vi "WPI_SolenoidSafetyError.vi"(0 "SolenoidDevRef":T1={"DevStatus"={"status"=FALSE, "code"=0, "source"=""}, "Pneumatics Control Module"=1, "Forward Solenoid Channel"=enum."Solenoid 0", "Reverse Solenoid Channel"=enum."Invalid"}) -> (4 "SolenoidDevRef 2":T1={"DevStatus"={"status"=FALSE, "code"=0, "source"=""}, "Pneumatics Control Module"=1, "Forward Solenoid Channel"=enum."Solenoid 0", "Reverse Solenoid Channel"=enum."Invalid"})   [LabVIEW 2017]
doc: "This subVI does two things:\n1. It builds up output specific information to help locate the problem.\n2. It calls the FRC Build Error, so all the information gets passed to the Driver Station."
uses:
  <vilib>/Rock Robotics/WPI/Solenoid/WPI_SolenoidDevRef.ctl
  <vilib>/Rock Robotics/WPI/Solenoid/WPI_SolenoidChannel.ctl
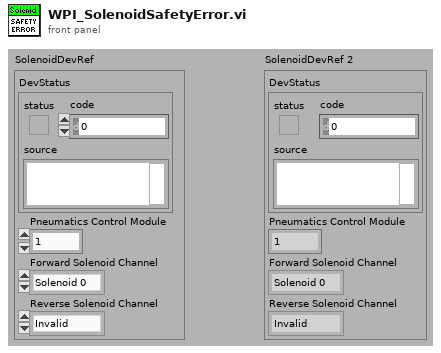
[diagram p1: front panel]
types:
  T1 = typedef "WPI_SolenoidDevRef.ctl" = cluster{"DevStatus":errorcluster, "Pneumatics Control Module":u8, "Forward Solenoid Channel":T2, "Reverse Solenoid Channel":T2}
  T2 = typedef "WPI_SolenoidChannel.ctl" = enum8{"Solenoid 0", "Solenoid 1", "Solenoid 2", "Solenoid 3", "Solenoid 4", "Solenoid 5", "Solenoid 6", "Solenoid 7", "Invalid"}
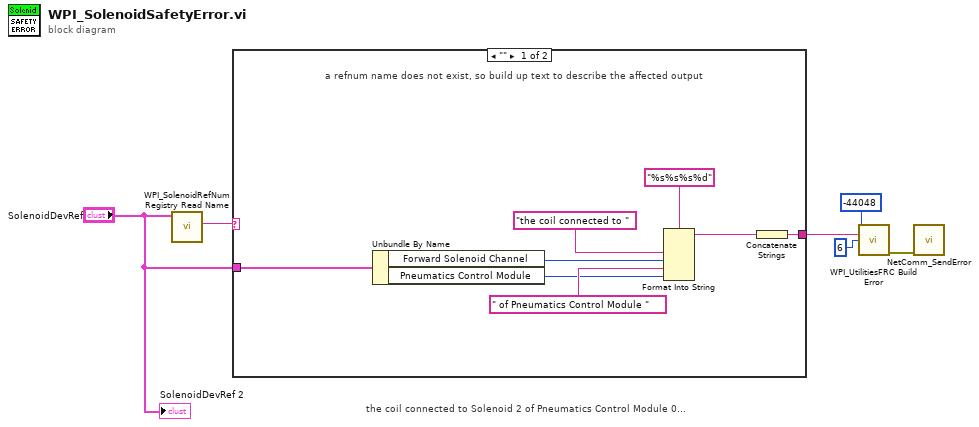
[diagram p0: block diagram]
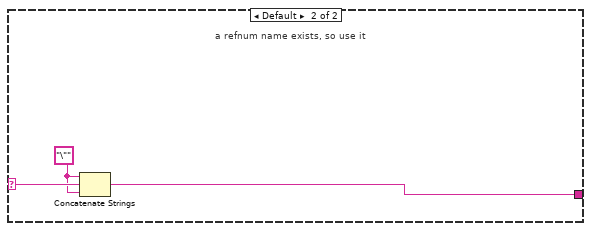
[diagram p2: hidden frame]
diagram:
  # "the coil connected to Solenoid 2 of Pneumatics Control Module 0..."
  n1 = call <vilib>:"WPI_SolenoidRefNum Registry Read Name.vi"("SolenoidDevRef"="SolenoidDevRef") -> ("refnum name"=w4:string)  [unwired: 1 in, 9 out]
  n2 = case shown="\"\"" w4 {
    selector: w4 -> [_ w17]
    tunnel: [w13 w16] -> w3
    tunnel: "SolenoidDevRef" -> [w12 _]
    frame "" {
      # "a refnum name does not exist, so build up text to describe the affected output"
      n3 = Unbundle By Name(w12) -> ("Forward Solenoid Channel"=w9:T2, "Pneumatics Control Module"=w7:u8)
      n4 = Format Into String(format string="%s%s%s%d", "the coil connected to " ("format string"), w9, " of Pneumatics Control Module " ("format string"), w7) -> (resulting string=w14:string)  [unwired: 2 in, 1 out]
      n5 = Concatenate Strings(w14) -> (w13:string)
    }
    frame Default {
      w15 = "\"" ("string")
      # "a refnum name exists, so use it"
      n6 = Concatenate Strings(w15, w17, w15) -> (w16:string)
    }
  }
  n7 = call <vilib>:"WPI_UtilitiesFRC Build Error.vi"("error code"=-44048 ("code"), "extra error text"=w3, "chain levels to remove (1)"=6) -> ("error out"=w1:errorcluster)  [unwired: 3 in, 9 out]
  n8 = call <vilib>:"NetComm_SendError.vi"("error in (no error)"=w1) -> ()  [unwired: 11 in]
  "SolenoidDevRef 2" <- "SolenoidDevRef"
